vi "STATUS.vi"(8 "error in (no error)":errorcluster, 11 "S4GUI in":refnum<class "S4GUI.lvclass">) -> (0 "error out":errorcluster, 3 "S4GUI out":refnum<class "S4GUI.lvclass">)   [LabVIEW 2018, in "S4GUI.lvclass"]
uses:
  S4GUI.lvclass
  S4GUI.lvclass/S4GUI.ctl
  Instrument/Instrument.lvclass/Instrument.ctl
  Device/Optics/Opt_Selector/Opt_Selector.lvclass
  Acquisition/Acquisition.lvclass
  Channel/Channel.lvclass
  StateMachine/State Machine.lvclass
  Instrument/Instrument.lvclass
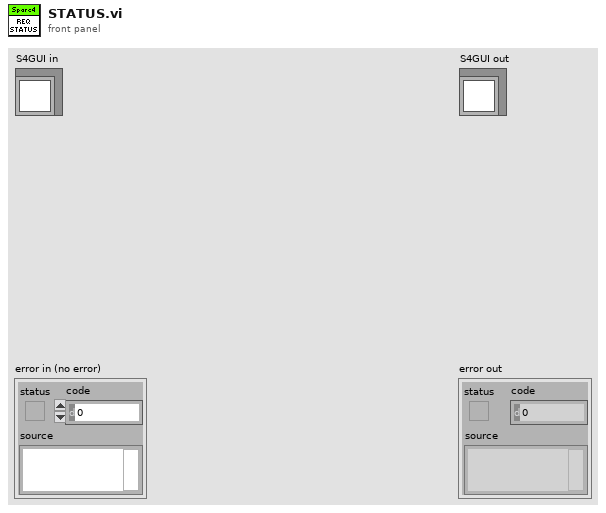
[diagram p1: front panel]
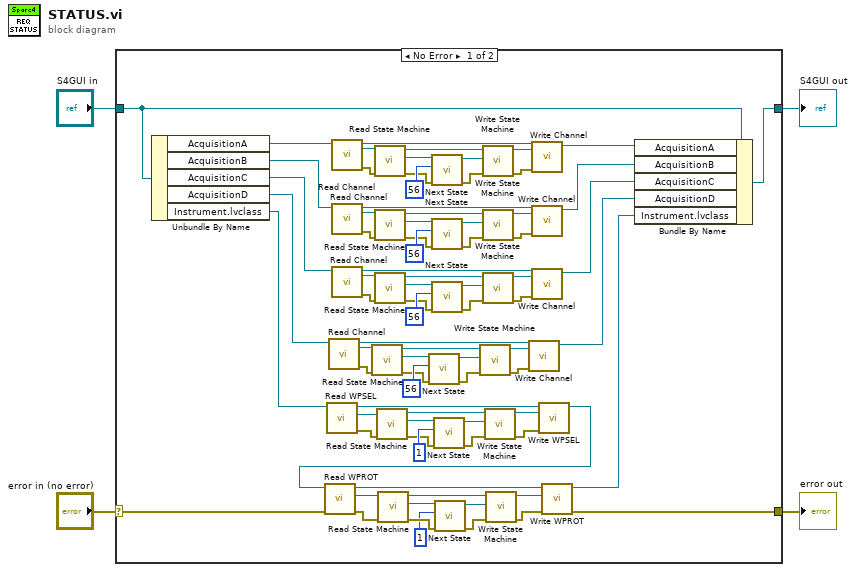
[diagram p0: block diagram]
diagram:
  n1 = case shown="No Error" "error in (no error)" {
    selector: "error in (no error)" -> [w47 w87]
    tunnel: [w46 w87] -> w3
    tunnel: [w84 w86] -> w1
    tunnel: "S4GUI in" -> [w85 w86]
    frame No Error {
      n2 = Unbundle By Name(w85) -> ("AcquisitionA"=w83:refnum<class "Acquisition.lvclass">, "AcquisitionB"=w12:refnum<class "Acquisition.lvclass">, "AcquisitionC"=w10:refnum<class "Acquisition.lvclass">, "AcquisitionD"=w8:refnum<class "Acquisition.lvclass">, "Instrument.lvclass"=w6:refnum<class "Instrument.lvclass">)
      n3 = call "Read WPSEL.vi"("Instrument in"=w6) -> ("error out"=w59:errorcluster, "Opt_Selector.lvclass"=w57:refnum<class "Opt_Selector.lvclass">, "Instrument out"=w60:refnum<class "Instrument.lvclass">)  [unwired: 8 in]
      n4 = call-dynamic "Read Channel.vi"("Acquisition in"=w8) -> ("error out"=w16:errorcluster, "Channel.lvclass"=w22:refnum<class "Channel.lvclass">, "Acquisition out"=w23:refnum<class "Acquisition.lvclass">)  [unwired: 8 in]
      n5 = call-dynamic "Read Channel.vi"("Acquisition in"=w83) -> ("error out"=w74:errorcluster, "Channel.lvclass"=w81:refnum<class "Channel.lvclass">, "Acquisition out"=w82:refnum<class "Acquisition.lvclass">)  [unwired: 8 in]
      n6 = call-dynamic "Read Channel.vi"("Acquisition in"=w12) -> ("error out"=w38:errorcluster, "Channel.lvclass"=w44:refnum<class "Channel.lvclass">, "Acquisition out"=w45:refnum<class "Acquisition.lvclass">)  [unwired: 8 in]
      n7 = call-dynamic "Read Channel.vi"("Acquisition in"=w10) -> ("error out"=w27:errorcluster, "Channel.lvclass"=w33:refnum<class "Channel.lvclass">, "Acquisition out"=w34:refnum<class "Acquisition.lvclass">)  [unwired: 8 in]
      n8 = call-dynamic "Read State Machine.vi"("error in (no error)"=w16, "Device in"=w22) -> ("error out"=w15:errorcluster, "State Machine.lvclass"=w19:refnum<class "State Machine.lvclass">, "Device out"=w21:refnum<class "Channel.lvclass">)  [unwired: 7 in]
      n9 = call-dynamic "Read State Machine.vi"("error in (no error)"=w74, "Device in"=w81) -> ("error out"=w73:errorcluster, "State Machine.lvclass"=w77:refnum<class "State Machine.lvclass">, "Device out"=w80:refnum<class "Channel.lvclass">)  [unwired: 7 in]
      n10 = call-dynamic "Read State Machine.vi"("error in (no error)"=w38, "Device in"=w44) -> ("error out"=w37:errorcluster, "State Machine.lvclass"=w41:refnum<class "State Machine.lvclass">, "Device out"=w43:refnum<class "Channel.lvclass">)  [unwired: 7 in]
      n11 = call-dynamic "Read State Machine.vi"("error in (no error)"=w27, "Device in"=w33) -> ("error out"=w26:errorcluster, "State Machine.lvclass"=w30:refnum<class "State Machine.lvclass">, "Device out"=w32:refnum<class "Channel.lvclass">)  [unwired: 7 in]
      n12 = call-dynamic "Read State Machine.vi"("error in (no error)"=w59, "Device in"=w57) -> ("error out"=w67:errorcluster, "State Machine.lvclass"=w70:refnum<class "State Machine.lvclass">, "Device out"=w56:refnum<class "Opt_Selector.lvclass">)  [unwired: 7 in]
      n13 = call "Next State.vi"("error in (no error)"=w15, "New_State"=56, "State Machine in"=w19) -> ("error out"=w14:errorcluster, "State Machine out"=w18:refnum<class "State Machine.lvclass">)  [unwired: 7 in]
      n14 = call "Next State.vi"("error in (no error)"=w73, "New_State"=56, "State Machine in"=w77) -> ("error out"=w72:errorcluster, "State Machine out"=w76:refnum<class "State Machine.lvclass">)  [unwired: 7 in]
      n15 = call "Next State.vi"("error in (no error)"=w37, "New_State"=56, "State Machine in"=w41) -> ("error out"=w36:errorcluster, "State Machine out"=w40:refnum<class "State Machine.lvclass">)  [unwired: 7 in]
      n16 = call "Next State.vi"("error in (no error)"=w26, "New_State"=56, "State Machine in"=w30) -> ("error out"=w25:errorcluster, "State Machine out"=w29:refnum<class "State Machine.lvclass">)  [unwired: 7 in]
      n17 = call "Next State.vi"("error in (no error)"=w67, "New_State"=1, "State Machine in"=w70) -> ("error out"=w66:errorcluster, "State Machine out"=w69:refnum<class "State Machine.lvclass">)  [unwired: 7 in]
      n18 = call-dynamic "Write State Machine.vi"("error in (no error)"=w14, "State Machine.lvclass"=w18, "Device in"=w21) -> ("error out"=w13:errorcluster, "Device out"=w20:refnum<class "Channel.lvclass">)  [unwired: 7 in]
      n19 = call-dynamic "Write State Machine.vi"("error in (no error)"=w72, "State Machine.lvclass"=w76, "Device in"=w80) -> ("error out"=w71:errorcluster, "Device out"=w79:refnum<class "Channel.lvclass">)  [unwired: 7 in]
      n20 = call-dynamic "Write State Machine.vi"("error in (no error)"=w36, "State Machine.lvclass"=w40, "Device in"=w43) -> ("error out"=w35:errorcluster, "Device out"=w42:refnum<class "Channel.lvclass">)  [unwired: 7 in]
      n21 = call-dynamic "Write State Machine.vi"("error in (no error)"=w25, "State Machine.lvclass"=w29, "Device in"=w32) -> ("error out"=w24:errorcluster, "Device out"=w31:refnum<class "Channel.lvclass">)  [unwired: 7 in]
      n22 = call-dynamic "Write State Machine.vi"("error in (no error)"=w66, "State Machine.lvclass"=w69, "Device in"=w56) -> ("error out"=w58:errorcluster, "Device out"=w55:refnum<class "Opt_Selector.lvclass">)  [unwired: 7 in]
      n23 = call-dynamic "Write Channel.vi"("error in (no error)"=w13, "Channel.lvclass"=w20, "Acquisition in"=w23) -> ("Acquisition out"=w7:refnum<class "Acquisition.lvclass">)  [unwired: 7 in, 1 out]
      n24 = call-dynamic "Write Channel.vi"("error in (no error)"=w71, "Channel.lvclass"=w79, "Acquisition in"=w82) -> ("Acquisition out"=w78:refnum<class "Acquisition.lvclass">)  [unwired: 7 in, 1 out]
      n25 = call-dynamic "Write Channel.vi"("error in (no error)"=w35, "Channel.lvclass"=w42, "Acquisition in"=w45) -> ("Acquisition out"=w11:refnum<class "Acquisition.lvclass">)  [unwired: 7 in, 1 out]
      n26 = call-dynamic "Write Channel.vi"("error in (no error)"=w24, "Channel.lvclass"=w31, "Acquisition in"=w34) -> ("Acquisition out"=w9:refnum<class "Acquisition.lvclass">)  [unwired: 7 in, 1 out]
      n27 = call "Write WPSEL.vi"("error in (no error)"=w58, "Opt_Selector.lvclass"=w55, "Instrument in"=w60) -> ("Instrument out"=w54:refnum<class "Instrument.lvclass">)  [unwired: 7 in, 1 out]
      n28 = call "Read WPROT.vi"("error in (no error)"=w47, "Instrument in"=w54) -> ("error out"=w53:errorcluster, "Opt_Selector.lvclass"=w50:refnum<class "Opt_Selector.lvclass">, "Instrument out"=w51:refnum<class "Instrument.lvclass">)  [unwired: 7 in]
      n29 = call-dynamic "Read State Machine.vi"("error in (no error)"=w53, "Device in"=w50) -> ("error out"=w64:errorcluster, "State Machine.lvclass"=w61:refnum<class "State Machine.lvclass">, "Device out"=w49:refnum<class "Opt_Selector.lvclass">)  [unwired: 7 in]
      n30 = call "Next State.vi"("error in (no error)"=w64, "New_State"=1, "State Machine in"=w61) -> ("error out"=w65:errorcluster, "State Machine out"=w62:refnum<class "State Machine.lvclass">)  [unwired: 7 in]
      n31 = call-dynamic "Write State Machine.vi"("error in (no error)"=w65, "State Machine.lvclass"=w62, "Device in"=w49) -> ("error out"=w52:errorcluster, "Device out"=w48:refnum<class "Opt_Selector.lvclass">)  [unwired: 7 in]
      n32 = call "Write WPROT.vi"("error in (no error)"=w52, "Opt_Selector.lvclass"=w48, "Instrument in"=w51) -> ("error out"=w46:errorcluster, "Instrument out"=w5:refnum<class "Instrument.lvclass">)  [unwired: 7 in]
      n33 = Bundle By Name(cluster=w85, "AcquisitionA"=w78, "AcquisitionB"=w11, "AcquisitionC"=w9, "AcquisitionD"=w7, "Instrument.lvclass"=w5) -> (w84:refnum<class "S4GUI.lvclass">)
    }
    frame Error {
    }
  }
  "error out" <- w3
  "S4GUI out" <- w1
